vi "get-tool-last-line.vi"(8 "Tool array in":T1[](array[typedef]), 11 "tool# or drive subsystem name":string) -> (0 "Found?":bool, 3 "Last line sent":i32)   [LabVIEW 2017]
uses:
  type-defs/tool-call-tracker.ctl
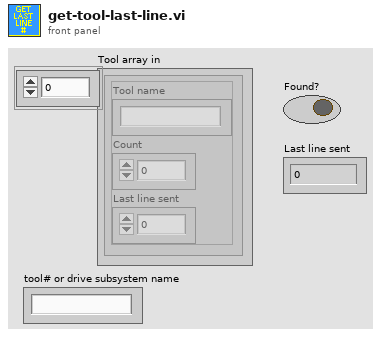
[diagram p1: front panel]
types:
  T1 = typedef "tool-call-tracker.ctl" = cluster{"Tool name":string, "Count":i32, "Last line sent":i32}
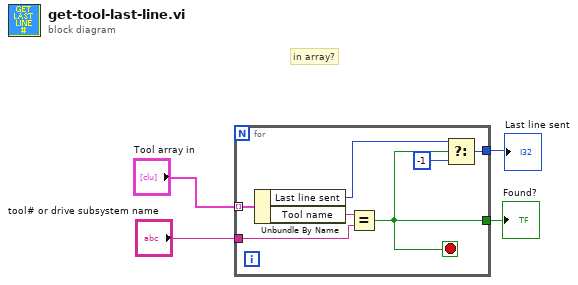
[diagram p0: block diagram]
diagram:
  # "in array?"
  n1 = for {
    tunnel: "Tool array in" -> [w11] mode=indexing
    tunnel: "tool# or drive subsystem name" -> [w9]
    tunnel: [w6] -> w2
    tunnel: [w8] -> w1
    stop <- w6 stop-if-true
    n2 = Unbundle By Name(w11) -> ("Last line sent"=w7:i32, "Tool name"=w10:string)
    n3 = Equal?(x=w10, y=w9) -> (x = y?=w6:bool)
    n4 = Select(t=w7, s=w6, f=-1) -> (s? t:f=w8:i32)
  }
  "Last line sent" <- w1
  "Found?" <- w2
